vi "Build Wiring Spec.vi"(8 "error in (no error)":errorcluster, 11 "CS++Actor in":refnum<class "CS++Actor.lvclass">) -> (0 "error out":errorcluster, 2 "Wiring Spec":T1, 3 "CS++Actor out":refnum<class "CS++Actor.lvclass">)   [LabVIEW 2014, in "CS++Actor.lvlib" / "CS++Actor.lvclass"]
doc: "Create the Wiring Spec of the original public Vi."
uses:
  CS++Actor.lvclass
  CS++Actor.lvclass/CS++Actor.ctl
  <vilib>/Utility/VariantDataType/VariantType.lvlib
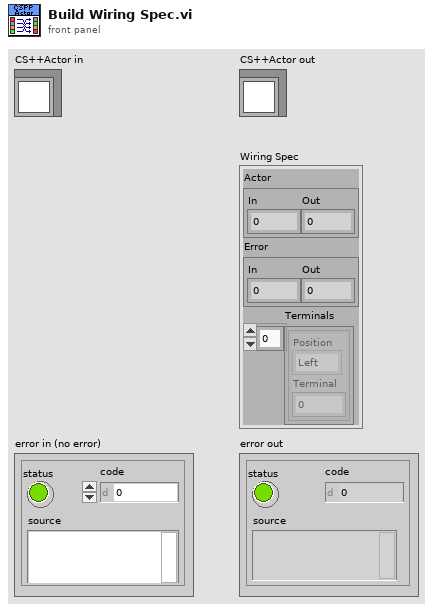
[diagram p1: front panel]
types:
  T1 = cluster{"Actor":cluster{"In":i32, "Out":i32}, "Error":cluster{"In":i32, "Out":i32}, "Terminals":cluster{"Position":enum16{"Left", "Top", "Bottom", "Right"}, "Terminal":i32}[]}
  T2 = cluster{"Actor":cluster{"In":i32, "Out":i32}, "Error":cluster{"In":i32, "Out":i32}, "Left":cluster{"Position":i16, "Terminal":i32}[], "Bottom":cluster{"Position":i16, "Terminal":i32}[], "Right":cluster{"Position":i16, "Terminal":i32}[], "Top":cluster{"Position":i16, "Terminal":i32}[]}
  T3 = enum16{"Invalid Wire Rule", "Required", "Recommended", "Optional", "Dynamic Dispatch"}[]
  T4 = typedef "LVRectTypeDef.ctl" = cluster{"Left":i16, "Top":i16, "Right":i16, "Bottom":i16}
  T5 = cluster{"Position":enum16{"Left", "Top", "Bottom", "Right"}, "Terminal":i32}
  T6 = cluster{"Position":enum16{"Left", "Top", "Bottom", "Right"}, "Terminal":i32}[]
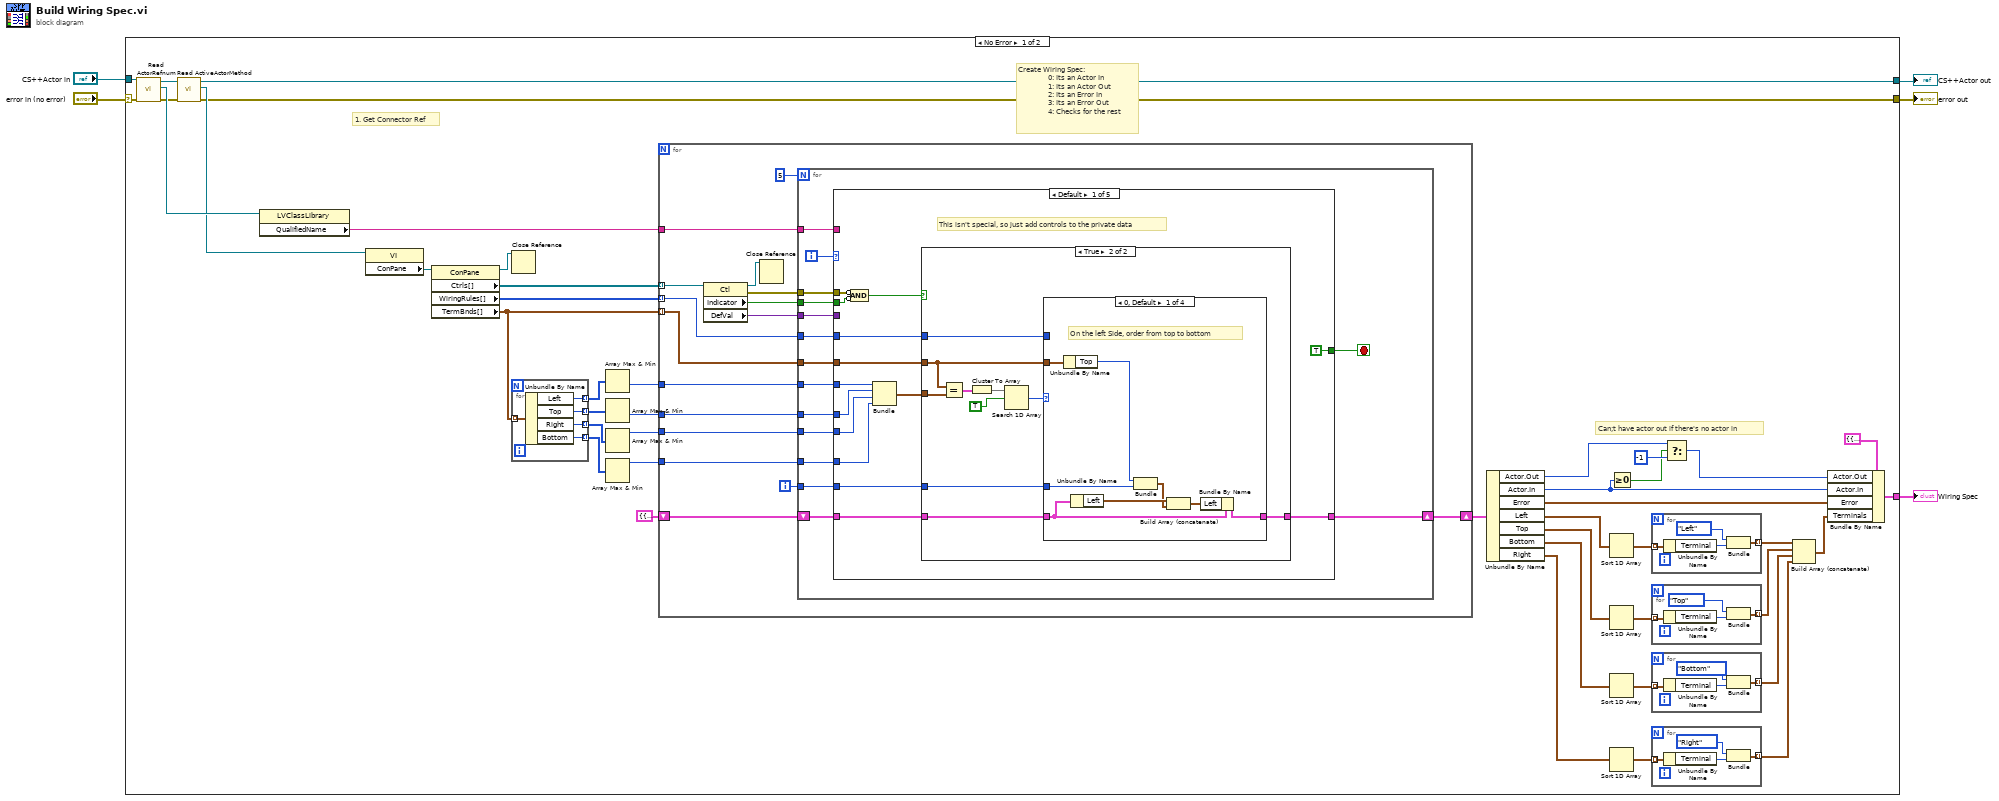
[diagram p0: block diagram]
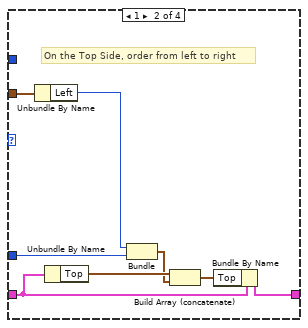
[diagram p3: hidden frame]
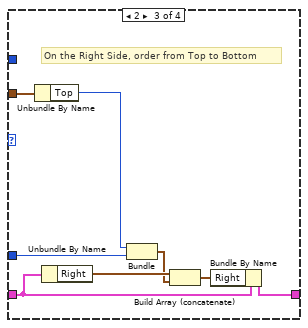
[diagram p4: hidden frame]
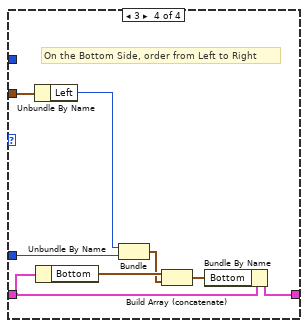
[diagram p5: hidden frame]
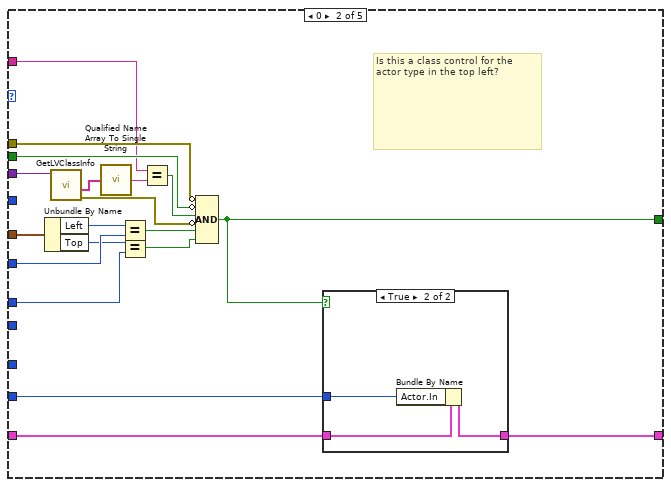
[diagram p6: hidden frame]
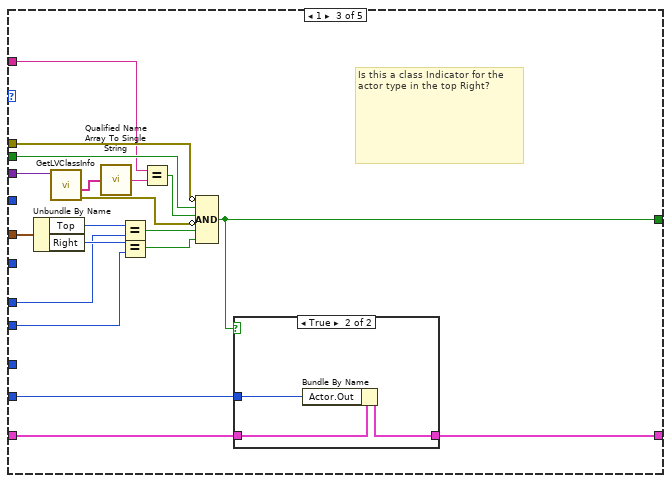
[diagram p8: hidden frame]
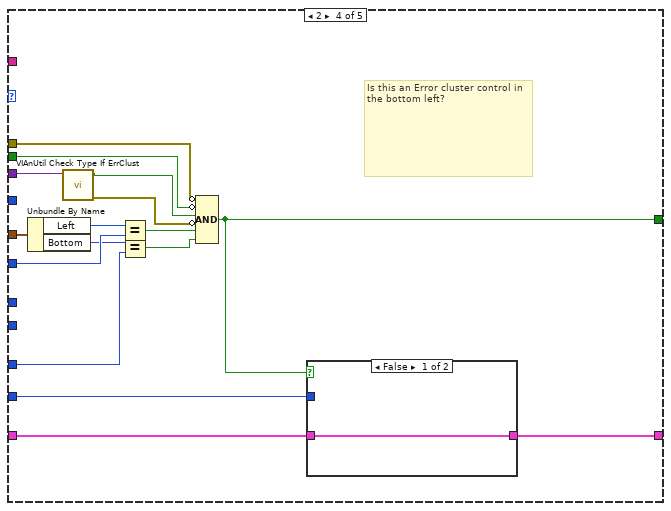
[diagram p10: hidden frame]
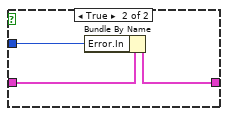
[diagram p11: hidden frame]
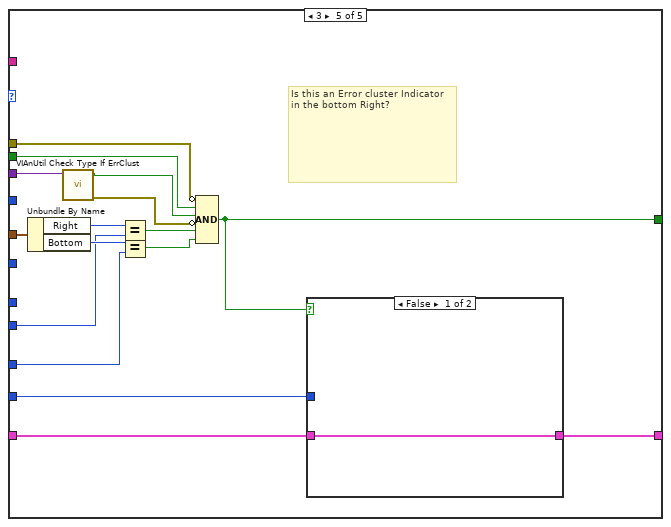
[diagram p12: hidden frame]
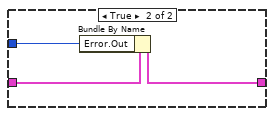
[diagram p13: hidden frame]
diagram:
  n1 = case shown="No Error" "error in (no error)" {
    selector: "error in (no error)" -> [w6 w246]
    tunnel: [w27 _] -> w5
    tunnel: "CS++Actor in" -> [w13 w247]
    tunnel: [w8 w246] -> w3
    tunnel: [w7 w247] -> w2
    frame No Error {
      # "Create Wiring Spec:\n               0: Its an Actor In\n               1: Its an Actor Out\n               2: Its an Error In\n               3: Its an Error Out \n               4: Checks for the rest"
      # "1. Get Connector Ref"
      # "Can;t have actor out if there's no actor in"
      n2 = call "Read ActorRefnum.vi"("error in (no error)"=w6, "CS++Actor in"=w13) -> ("error out"=w10:errorcluster, "ActorRefnum"=w12:refnum<vi>, "CS++Actor out"=w11:refnum<class "CS++Actor.lvclass">)  [unwired: 7 in]
      n3 = call "Read ActiveActorMethod.vi"("error in (no error)"=w10, "CS++Actor in"=w11) -> ("error out"=w8:errorcluster, "ActiveActorMethod"=w9:refnum<vi>, "CS++Actor out"=w7:refnum<class "CS++Actor.lvclass">)  [unwired: 7 in]
      n4 = property class="LVClassLibrary"(reference=w12) -> ("QualifiedName"=w14:string)  [unwired: 1 in, 2 out]
      n5 = property class="VI"(reference=w9) -> ("ConPane"=w50:refnum<vi>)  [unwired: 1 in, 2 out]
      n6 = property class="ConPane"(reference=w50) -> (reference out=w39:refnum<vi>, "Ctrls[]"=w49:refnum<vi>[], "WiringRules[]"=w26:T3, "TermBnds[]"=w48:T4[])  [unwired: 1 in, 1 out]
      n7 = Close Reference(reference=w39) -> ()  [unwired: 1 in, 1 out]
      n8 = for {
        tunnel: w48 -> [w71] mode=indexing
        tunnel: [w70] -> w47 mode=indexing
        tunnel: [w69] -> w46 mode=indexing
        tunnel: [w68] -> w45 mode=indexing
        tunnel: [w67] -> w44 mode=indexing
        n9 = Unbundle By Name(w71) -> ("Left"=w70:i16, "Top"=w69:i16, "Right"=w68:i16, "Bottom"=w67:i16)
      }
      n10 = Array Max & Min(array=w47) -> (min value=w43:i16)  [unwired: 3 out]
      n11 = Array Max & Min(array=w46) -> (min value=w42:i16)  [unwired: 3 out]
      n12 = Array Max & Min(array=w45) -> (max value=w41:i16)  [unwired: 3 out]
      n13 = Array Max & Min(array=w44) -> (max value=w40:i16)  [unwired: 3 out]
      n14 = for {
        tunnel: w49 -> [w87] mode=indexing
        tunnel: w48 -> [w85] mode=indexing
        tunnel: w43 -> [w84]
        tunnel: w42 -> [w83]
        tunnel: w41 -> [w76]
        tunnel: w40 -> [w77]
        tunnel: w14 -> [w79]
        shift-right: [w73] -> w37
        shift-left: T2 {"Actor"={"In"=-1, "Out"=-1}, "Error"={"In"=-1, "Out"=-1}, "Left"=[], "Bottom"=[], "Right"=[], "Top"=[]} -> [w74]
        tunnel: w26 -> [w72] mode=indexing
        i -> [w78]
        # "Find Top Left, Bottom left controls AND\nTop Right and bottom right Indicators"
        n15 = property class="Ctl"(reference=w87) -> (reference out=w75:refnum<vi>, error out=w82:errorcluster, "Indicator"=w81:bool, "DefVal"=w80:variant)  [unwired: 1 in]
        n16 = Close Reference(reference=w75) -> ()  [unwired: 1 in, 1 out]
        n17 = for {
          N: 5 -> [_]
          tunnel: w85 -> [w101]
          shift-right: [w92] -> w73
          shift-left: w74 -> [w100]
          tunnel: w84 -> [w99]
          tunnel: w83 -> [w98]
          tunnel: w82 -> [w97]
          tunnel: w81 -> [w96]
          tunnel: w80 -> [w95]
          tunnel: w79 -> [w94]
          tunnel: w78 -> [w93]
          tunnel: w77 -> [w91]
          tunnel: w76 -> [w90]
          tunnel: w72 -> [w88]
          i -> [w102]
          stop <- w89 stop-if-true
          n18 = case shown="Default" w102 {
            tunnel: w101 -> [w109 w178 w201 w221 w241]
            tunnel: w100 -> [w116 w163 w188 w207 w227]
            tunnel: w99 -> [w108 w176 _ w219 _]
            tunnel: w98 -> [w107 w174 w186 _ _]
            tunnel: w97 -> [w114 w173 w198 w217 w238]
            tunnel: w96 -> [w113 w172 w197 w216 w237]
            tunnel: w95 -> [_ w168 w193 w212 w233]
            tunnel: w94 -> [_ w165 w190 _ _]
            tunnel: w93 -> [w111 w162 w187 w213 w234]
            tunnel: [w115 w160 w183 w206 w226] -> w92
            tunnel: w91 -> [w105 _ _ w209 w230]
            tunnel: w90 -> [w106 _ w185 _ w229]
            tunnel: [TRUE w161 w184 w208 w228] -> w89
            tunnel: w88 -> [w103 _ _ _ _]
            frame Default {
              # "This isn't special, so just add controls to the private data"
              n19 = Compound Arithmetic op=AND(invert w114, invert w113) -> (w112:bool)
              n20 = Bundle(w108, w107, w106, w105) -> (w104:cluster{i16, i16, i16, i16})  [unwired: 1 in]
              n21 = case shown="True" w112 {
                tunnel: w116 -> [w117 w121]
                tunnel: [w117 w119] -> w115
                tunnel: w111 -> [_ w120]
                tunnel: w109 -> [_ w122]
                tunnel: w104 -> [_ w127]
                tunnel: w103 -> [_ w118]
                frame False {
                }
                frame True {
                  n22 = Equal?(x=w122, y=w127) -> (x = y?=w126:cluster{bool, bool, bool, bool})
                  n23 = Cluster To Array(cluster=w126) -> (array=w125:bool[])
                  n24 = Search 1D Array(1D array=w125, element=TRUE) -> (index of element=w123:i32)  [unwired: 1 in]
                  n25 = case shown="0, Default" w123 {
                    tunnel: w122 -> [w135 w143 w151 w159]
                    tunnel: w121 -> [w132 w140 w148 w156]
                    tunnel: w120 -> [w133 w141 w149 w157]
                    tunnel: [w129 w137 w145 w153] -> w119
                    tunnel: w118 -> [_ _ _ _]
                    frame 0, Default {
                      # "On the left Side, order from top to bottom"
                      n26 = Unbundle By Name(w135) -> ("Top"=w134:i16)
                      n27 = Unbundle By Name(w132) -> ("Left"=w131:cluster{"Position":i16, "Terminal":i32}[])
                      n28 = Bundle("Top"=w134, w133) -> (w130:cluster{"Top":i16, i32})  [unwired: 1 in]
                      n29 = Build Array (concatenate)(w131, w130) -> (w128:cluster{"Top":i16, "Terminal":i32}[])
                      n30 = Bundle By Name(cluster=w132, "Left"=w128) -> (w129:T2)
                    }
                    frame 1 {
                      # "On the Top Side, order from left to right"
                      n31 = Unbundle By Name(w143) -> ("Left"=w142:i16)
                      n32 = Unbundle By Name(w140) -> ("Top"=w139:cluster{"Position":i16, "Terminal":i32}[])
                      n33 = Bundle("Left"=w142, w141) -> (w138:cluster{"Left":i16, i32})  [unwired: 1 in]
                      n34 = Build Array (concatenate)(w139, w138) -> (w136:cluster{"Left":i16, "Terminal":i32}[])
                      n35 = Bundle By Name(cluster=w140, "Top"=w136) -> (w137:T2)
                    }
                    frame 2 {
                      # "On the Right Side, order from Top to Bottom"
                      n36 = Unbundle By Name(w151) -> ("Top"=w150:i16)
                      n37 = Unbundle By Name(w148) -> ("Right"=w147:cluster{"Position":i16, "Terminal":i32}[])
                      n38 = Bundle("Top"=w150, w149) -> (w146:cluster{"Top":i16, i32})  [unwired: 1 in]
                      n39 = Build Array (concatenate)(w147, w146) -> (w144:cluster{"Top":i16, "Terminal":i32}[])
                      n40 = Bundle By Name(cluster=w148, "Right"=w144) -> (w145:T2)
                    }
                    frame 3 {
                      # "On the Bottom Side, order from Left to Right"
                      n41 = Unbundle By Name(w159) -> ("Left"=w158:i16)
                      n42 = Unbundle By Name(w156) -> ("Bottom"=w155:cluster{"Position":i16, "Terminal":i32}[])
                      n43 = Bundle("Left"=w158, w157) -> (w154:cluster{"Left":i16, i32})  [unwired: 1 in]
                      n44 = Build Array (concatenate)(w155, w154) -> (w152:cluster{"Left":i16, "Terminal":i32}[])
                      n45 = Bundle By Name(cluster=w156, "Bottom"=w152) -> (w153:T2)
                    }
                  }
                }
              }
            }
            frame 0 {
              # "Is this a class control for the actor type in the top left?"
              # "Top Left Actor Class Ctrl?"
              n46 = Unbundle By Name(w178) -> ("Left"=w177:i16, "Top"=w175:i16)
              n47 = call <vilib>:"GetLVClassInfo.vi"("Variant"=w168) -> ("error out"=w167:errorcluster, "Fully Qualified LV Class Name"=w169:string[])  [unwired: 8 in, 1 out]
              n48 = call <vilib>:"Qualified Name Array To Single String.vi"("Fully Qualified Array"=w169) -> ("Fully Qualified String"=w166:string)
              n49 = Equal?(x=w177, y=w176) -> (x = y?=w171:bool)
              n50 = Equal?(x=w175, y=w174) -> (x = y?=w170:bool)
              n51 = Equal?(x=w165, y=w166) -> (x = y?=w164:bool)
              n52 = Compound Arithmetic op=AND(invert w173, invert w172, w164, invert w167, w171, w170) -> (w161:bool)
              n53 = case shown="True" w161 {
                tunnel: w163 -> [w179 w180]
                tunnel: w162 -> [_ w181]
                tunnel: [w179 w182] -> w160
                frame False {
                }
                frame True {
                  n54 = Bundle By Name(cluster=w180, "Actor.In"=w181) -> (w182:T2)
                }
              }
            }
            frame 1 {
              # "Is this a class Indicator for the actor type in the top Right?"
              # "Top Left Actor Class Ctrl?"
              n55 = Unbundle By Name(w201) -> ("Top"=w200:i16, "Right"=w199:i16)
              n56 = call <vilib>:"GetLVClassInfo.vi"("Variant"=w193) -> ("error out"=w192:errorcluster, "Fully Qualified LV Class Name"=w194:string[])  [unwired: 8 in, 1 out]
              n57 = call <vilib>:"Qualified Name Array To Single String.vi"("Fully Qualified Array"=w194) -> ("Fully Qualified String"=w191:string)
              n58 = Equal?(x=w200, y=w186) -> (x = y?=w196:bool)
              n59 = Equal?(x=w199, y=w185) -> (x = y?=w195:bool)
              n60 = Equal?(x=w190, y=w191) -> (x = y?=w189:bool)
              n61 = Compound Arithmetic op=AND(invert w198, w197, w189, invert w192, w196, w195) -> (w184:bool)
              n62 = case shown="True" w184 {
                tunnel: w188 -> [w202 w203]
                tunnel: w187 -> [_ w204]
                tunnel: [w202 w205] -> w183
                frame False {
                }
                frame True {
                  n63 = Bundle By Name(cluster=w203, "Actor.Out"=w204) -> (w205:T2)
                }
              }
            }
            frame 2 {
              # "Is this an Error cluster control in the bottom left?"
              # "Top Left Actor Class Ctrl?"
              n64 = Unbundle By Name(w221) -> ("Left"=w220:i16, "Bottom"=w218:i16)
              n65 = call <vilib>:"VIAnUtil Check Type If ErrClust.vi"("Data In"=w212) -> ("error out"=w211:errorcluster, "IsErrClust?"=w210:bool)  [unwired: 9 in]
              n66 = Equal?(x=w220, y=w219) -> (x = y?=w215:bool)
              n67 = Equal?(x=w218, y=w209) -> (x = y?=w214:bool)
              n68 = Compound Arithmetic op=AND(invert w217, invert w216, w210, invert w211, w215, w214) -> (w208:bool)
              n69 = case shown="False" w208 {
                tunnel: w213 -> [_ w224]
                tunnel: [w222 w225] -> w206
                tunnel: w207 -> [w222 w223]
                frame False {
                }
                frame True {
                  n70 = Bundle By Name(cluster=w223, "Error.In"=w224) -> (w225:T2)
                }
              }
            }
            frame 3 {
              # "Is this an Error cluster Indicator in the bottom Right?"
              # "Top Left Actor Class Ctrl?"
              n71 = Unbundle By Name(w241) -> ("Right"=w240:i16, "Bottom"=w239:i16)
              n72 = call <vilib>:"VIAnUtil Check Type If ErrClust.vi"("Data In"=w233) -> ("error out"=w232:errorcluster, "IsErrClust?"=w231:bool)  [unwired: 9 in]
              n73 = Equal?(x=w240, y=w229) -> (x = y?=w236:bool)
              n74 = Equal?(x=w239, y=w230) -> (x = y?=w235:bool)
              n75 = Compound Arithmetic op=AND(invert w238, w237, w231, invert w232, w236, w235) -> (w228:bool)
              n76 = case shown="False" w228 {
                tunnel: w234 -> [_ w244]
                tunnel: [w242 w245] -> w226
                tunnel: w227 -> [w242 w243]
                frame False {
                }
                frame True {
                  n77 = Bundle By Name(cluster=w243, "Error.Out"=w244) -> (w245:T2)
                }
              }
            }
          }
        }
      }
      n78 = Unbundle By Name(w37) -> ("Actor.Out"=w33:i32, "Actor.In"=w30:i32, "Error"=w35:cluster{"In":i32, "Out":i32}, "Left"=w29:cluster{"Position":i16, "Terminal":i32}[], "Top"=w22:cluster{"Position":i16, "Terminal":i32}[], "Bottom"=w21:cluster{"Position":i16, "Terminal":i32}[], "Right"=w20:cluster{"Position":i16, "Terminal":i32}[])
      n79 = Sort 1D Array(array=w29) -> (sorted array=w28:cluster{"Position":i16, "Terminal":i32}[])
      n80 = Sort 1D Array(array=w22) -> (sorted array=w25:cluster{"Position":i16, "Terminal":i32}[])
      n81 = Sort 1D Array(array=w21) -> (sorted array=w24:cluster{"Position":i16, "Terminal":i32}[])
      n82 = Sort 1D Array(array=w20) -> (sorted array=w23:cluster{"Position":i16, "Terminal":i32}[])
      n83 = Greater Or Equal To 0?(x=w30) -> (x >= 0?=w31:bool)
      n84 = for {
        tunnel: w28 -> [w66] mode=indexing
        tunnel: [w63] -> w19 mode=indexing
        n85 = Unbundle By Name(w66) -> ("Terminal"=w64:i32)
        n86 = Bundle("Position"=enum16{"Left", "Top", "Bottom", "Right"}."Left", "Terminal"=w64) -> (w63:T5)  [unwired: 1 in]
      }
      n87 = for {
        tunnel: w25 -> [w62] mode=indexing
        tunnel: [w59] -> w18 mode=indexing
        n88 = Unbundle By Name(w62) -> ("Terminal"=w60:i32)
        n89 = Bundle("Position"=enum16{"Left", "Top", "Bottom", "Right"}."Top", "Terminal"=w60) -> (w59:T5)  [unwired: 1 in]
      }
      n90 = for {
        tunnel: w24 -> [w58] mode=indexing
        tunnel: [w55] -> w17 mode=indexing
        n91 = Unbundle By Name(w58) -> ("Terminal"=w56:i32)
        n92 = Bundle("Position"=enum16{"Left", "Top", "Bottom", "Right"}."Bottom", "Terminal"=w56) -> (w55:T5)  [unwired: 1 in]
      }
      n93 = for {
        tunnel: w23 -> [w54] mode=indexing
        tunnel: [w51] -> w16 mode=indexing
        n94 = Unbundle By Name(w54) -> ("Terminal"=w52:i32)
        n95 = Bundle("Position"=enum16{"Left", "Top", "Bottom", "Right"}."Right", "Terminal"=w52) -> (w51:T5)  [unwired: 1 in]
      }
      n96 = Select(t=w33, s=w31, f=-1) -> (s? t:f=w34:i32)
      n97 = Build Array (concatenate)(w19, w18, w17, w16) -> (w15:T6)
      n98 = Bundle By Name(cluster=T1 {"Actor"={"In"=0, "Out"=0}, "Error"={"In"=0, "Out"=0}, "Terminals"=[]} ("Wiring Spec"), "Actor.Out"=w34, "Actor.In"=w30, "Error"=w35, "Terminals"=w15) -> (w27:T1)
    }
    frame Error {
    }
  }
  "Wiring Spec" <- w5
  "error out" <- w3
  "CS++Actor out" <- w2
